vi "Serial Daemon.vi"(8 "UUID":string, 9 "Data Model":refnum<class "Device Data Model.lvclass">, 10 "transmission data unit":refnum<class "Transmission Data Unit.lvclass">, 11 "serial slave":refnum<class "Serial Slave.lvclass">) -> ()   [LabVIEW 2012, in "Serial Slave.lvclass"]
uses:
  Serial Slave.lvclass
  Transmission Data Unit/Transmission Data Unit.lvclass
  Data Model/Device Data Model.lvclass
  daemon status.ctl
  Transmission Data Unit/Serial Interface/Serial Data Unit.lvclass
  Network Slave.lvclass/Network Slave.ctl
  Serial Slave.lvclass/Serial Slave.ctl
  <vilib>/Instr/_visa.llb/VISA Flush IO Buffer Mask.ctl
  Network Slave.lvclass
panel:
  in  "stop":bool
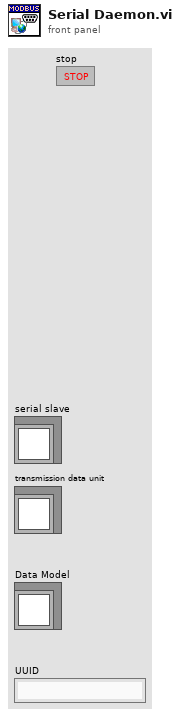
[diagram p1: front panel]
types:
  T1 = typedef "Network Slave.lvclass/daemon status.ctl" = enum16{"Not Started", "Running", "Error", "Stopped"}
  T2 = typedef "VISA Flush IO Buffer Mask.ctl" = u16
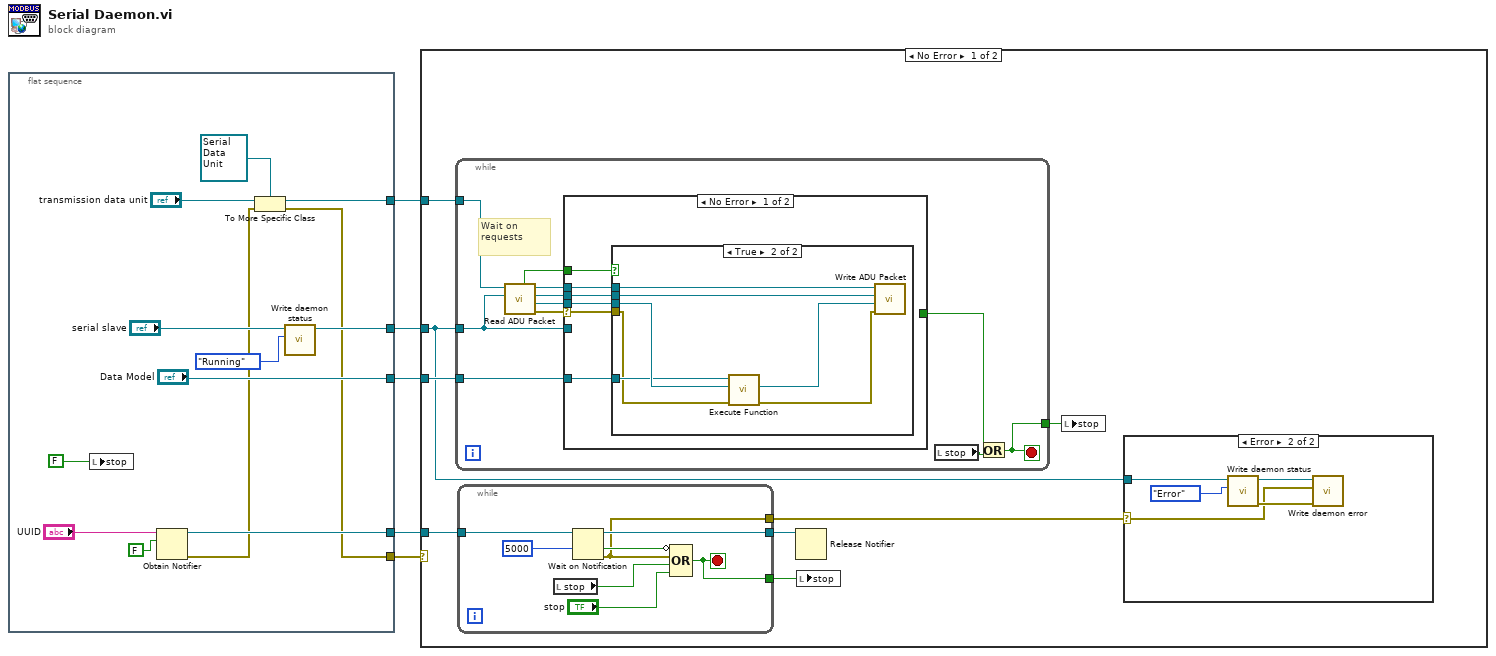
[diagram p0: block diagram]
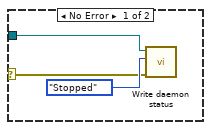
[diagram p2: hidden frame]
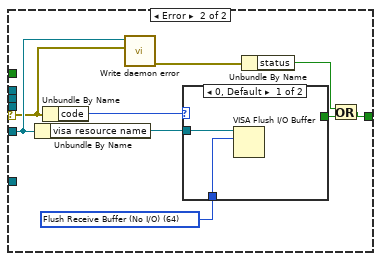
[diagram p4: hidden frame]
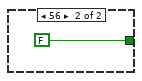
[diagram p5: hidden frame]
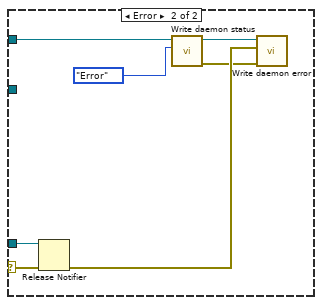
[diagram p6: hidden frame]
diagram:
  n1 = flat-sequence {
    tunnel: [w14] -> w1
    tunnel: [w10] -> w5
    tunnel: ["Data Model"] -> w4
    tunnel: [w8] -> w3
    tunnel: [w17] -> w2
    frame #0 {
      n2 = local write "stop"(FALSE ("stop")) -> ()
      n3 = Obtain Notifier(name (unnamed)="UUID", notification data type=FALSE) -> (notifier out=w17:refnum<notifier>, error out=w9:errorcluster)  [unwired: 2 in, 1 out]
      n4 = To More Specific Class(target class=refnum<class "Serial Data Unit.lvclass"> refnum ("Serial Data Unit"), reference="transmission data unit", error in=w9) -> (specific class reference=w10:refnum<class "Serial Data Unit.lvclass">, error out=w8:errorcluster)
      n5 = call "Write daemon status.vi"("daemon status"=daemon_status."Running", "Network Slave in"="serial slave") -> ("Network Slave out"=w14:refnum<class "Serial Slave.lvclass">)  [unwired: 8 in, 1 out]
    }
  }
  n6 = case shown="No Error" w3 {
    selector: w3 -> [_ w85]
    tunnel: w5 -> [w22 _]
    tunnel: w4 -> [w26 _]
    tunnel: w1 -> [w19 w83]
    tunnel: w2 -> [w25 w84]
    frame No Error {
      n7 = while {
        tunnel: w22 -> [w53]
        tunnel: w26 -> [w51]
        tunnel: w19 -> [w44]
        tunnel: [w48] -> w21
        stop <- w48 stop-if-true
        # "Wait on requests"
        n8 = call-dynamic "Read ADU Packet.vi"("protocol layer"=w44, "transmission data unit in"=w53) -> ("error out"=w52:errorcluster, "modbus data unit"=w46:refnum<class "Modbus Data Unit.lvclass">, "protocol layer out"=w45:refnum<class "Network Protocol.lvclass">, "transmission data unit out"=w50:refnum<class "Serial Data Unit.lvclass">, "PDU Valid?"=w43:bool)  [unwired: 5 in]
        n9 = case shown="No Error" w52 {
          selector: w52 -> [w55 w68]
          tunnel: w51 -> [w56 _]
          tunnel: w50 -> [w59 _]
          tunnel: [_ w71] -> w47
          tunnel: w46 -> [w58 _]
          tunnel: w45 -> [w57 _]
          tunnel: w44 -> [_ w69]
          tunnel: w43 -> [w54 _]
          frame No Error {
            n10 = case shown="True" w54 {
              tunnel: w59 -> [_ w66]
              tunnel: w58 -> [_ w65]
              tunnel: w57 -> [_ w62]
              tunnel: w56 -> [_ w61]
              tunnel: w55 -> [_ w60]
              frame False {
              }
              frame True {
                n11 = call-dynamic "Execute Function.vi"("error in"=w60, "modbus request"=w65, "device data model in"=w61) -> ("error out"=w63:errorcluster, "modbus response"=w64:refnum<class "Modbus Data Unit.lvclass">)  [unwired: 6 in, 1 out]
                n12 = call-dynamic "Write ADU Packet.vi"("error in"=w63, "modbus data unit"=w64, "protocol layer"=w62, "transmission data unit in"=w66) -> ()  [unwired: 5 in, 3 out]
              }
            }
          }
          frame Error {
            w73 = T2 64 items=["Flush Receive Buffer"=16, "Write Transmit Buffer to Device"=32, "Flush Receive Buffer (No I/O)"=64, "Flush Transmit Buffer"=128] ("Mask")
            n13 = Unbundle By Name(w69) -> ("visa resource name"=w74:refnum<visa-resource-name>)
            n14 = Unbundle By Name(w68) -> ("code"=w75:i32)
            n15 = call "Write daemon error.vi"("daemon error"=w68, "Network Slave in"=w69) -> ("error out"=w67:errorcluster)  [unwired: 8 in, 1 out]
            n16 = case shown="0, Default" w75 {
              tunnel: [_ FALSE ("stop")] -> w72
              tunnel: w74 -> [w77 _]
              tunnel: w73 -> [w76 _]
              frame 0, Default {
                n17 = VISA Flush I/O Buffer(VISA resource name=w77, mask (16)=w76) -> ()  [unwired: 1 in, 2 out]
              }
              frame 56 {
              }
            }
            n18 = Unbundle By Name(w67) -> ("status"=w70:bool)
            n19 = Or(x=w70, y=w72) -> (x .or. y?=w71:bool)
          }
        }
        n20 = local read "stop"() -> (w49:bool)
        n21 = Or(x=w47, y=w49) -> (x .or. y?=w48:bool)
      }
      n22 = while {
        tunnel: w25 -> [w41]
        tunnel: [w40] -> w23
        tunnel: [w36] -> w24
        tunnel: [w35] -> w20
        stop <- w36 stop-if-true
        n23 = local read "stop"() -> (w38:bool)
        n24 = Wait on Notification(notifier=w41, timeout in ms (-1)=5000) -> (notifier out=w40:refnum<notifier>, timed out?=w39:bool, error out=w35:errorcluster)  [unwired: 2 in, 1 out]
        n25 = Compound Arithmetic op=OR(invert w39, w35, w38, "stop") -> (w36:bool)
      }
      n26 = Release Notifier(notifier=w23) -> ()  [unwired: 2 in, 3 out]
      n27 = local write "stop"(w24) -> ()
      n28 = local write "stop"(w21) -> ()
      n29 = case shown="Error" w20 {
        selector: w20 -> [w28 w30]
        tunnel: w19 -> [w27 w32]
        frame No Error {
          n30 = call "Write daemon status.vi"("error in (no error)"=w28, "daemon status"=daemon_status."Stopped", "Network Slave in"=w27) -> ()  [unwired: 7 in, 2 out]
        }
        frame Error {
          n31 = call "Write daemon status.vi"("daemon status"=daemon_status."Error", "Network Slave in"=w32) -> ("error out"=w33:errorcluster, "Network Slave out"=w34:refnum<class "Serial Slave.lvclass">)  [unwired: 8 in]
          n32 = call "Write daemon error.vi"("error in (no error)"=w33, "daemon error"=w30, "Network Slave in"=w34) -> ()  [unwired: 7 in, 2 out]
        }
      }
    }
    frame Error {
      n33 = Release Notifier(notifier=w84, error in (no error)=w85) -> (error out=w80:errorcluster)  [unwired: 1 in, 2 out]
      n34 = call "Write daemon status.vi"("daemon status"=daemon_status."Error", "Network Slave in"=w83) -> ("error out"=w79:errorcluster, "Network Slave out"=w81:refnum<class "Serial Slave.lvclass">)  [unwired: 8 in]
      n35 = call "Write daemon error.vi"("error in (no error)"=w79, "daemon error"=w80, "Network Slave in"=w81) -> ()  [unwired: 7 in, 2 out]
    }
  }
